vi "Read Msg Output.vi"(10 "Msg Output":refnum<class "Msg Output.lvclass">) -> ()   [LabVIEW 2020, in "jettl.lvlib" / "Stopping jettl Msg.lvlib" / "Stopping Msg Output.lvlib"]
doc: "jettl 6.12.1.94\nNathan Davis - Nathan Davis\nCopyright (c) 2026, Nathan Davis\nMIT"
uses:
  Stopping Msg Output.lvlib
  Msg Output/Msg Output.lvclass
  Stopping Msg Output/Stopping Msg Output.lvclass
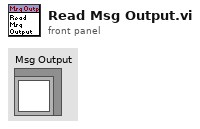
[diagram p1: front panel]
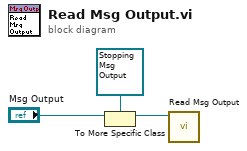
[diagram p0: block diagram]
diagram:
  n1 = To More Specific Class(target class=refnum<class "Stopping Msg Output.lvclass"> refnum ("_Template.lvlib:Templates.lvlib:TEMPLATE Msg.lvlib:TEMPLATE Msg Output.lvclass"), reference="Msg Output") -> (specific class reference=w1:refnum<class "Stopping Msg Output.lvclass">)  [unwired: 1 in, 1 out]
  n2 = call "Read Msg Output.vi"("Stopping Msg Output in"=w1) -> ()  [unwired: 11 in]
